vi "TimestampUpdate.vi"(10 "Timestamp":refnum<class "Timestamp.lvclass">, 11 "UserEvents":refnum<class "UserEvents.lvclass">) -> ()   [LabVIEW 2016]
uses:
  UserEvents/UserEvents.lvclass
  Common_RT_Timestamp/Timestamp/Timestamp.lvclass
  UserEvents/UserEvents.lvclass/UserEvents.ctl
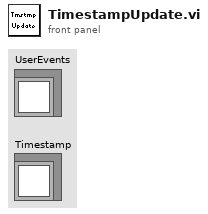
[diagram p1: front panel]
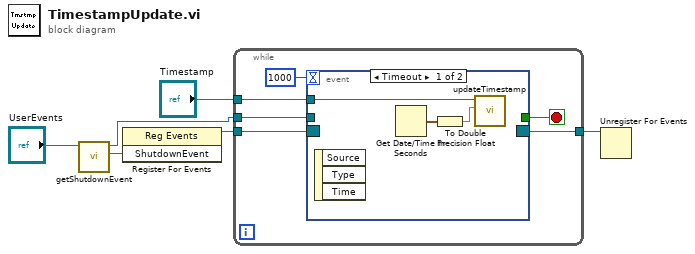
[diagram p0: block diagram]
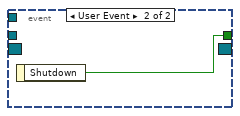
[diagram p2: hidden frame]
diagram:
  n1 = call "getShutdownEvent.vi"("UserEvents in"="UserEvents") -> ("ShutdownEvent"=w6:refnum<user-event>, "UserEvents out"=w4:refnum<class "UserEvents.lvclass">)  [unwired: 9 in]
  n2 = register-events(w6) -> (reference out=w5:refnum<event-registration>)  [unwired: 2 in, 1 out]
  n3 = while {
    tunnel: w5 -> [w11]
    tunnel: [w10] -> w3
    tunnel: w4 -> [w8]
    tunnel: "Timestamp" -> [w7]
    stop <- w9 stop-if-true
    n4 = event shown="[0] Timeout" {
      selector: w11 -> [_ _]
      dyn-events: [_ _] -> w10
      timeout: 1000 -> [_ _]
      tunnel: [_ w16] -> w9
      tunnel: w8 -> [_ _]
      tunnel: w7 -> [w15 _]
      event Timeout {
        n5 = event-data() -> ()  [unwired: 1 in, 3 out]
        n6 = Get Date/Time In Seconds() -> (seconds since 1Jan1904=w14:timestamp)
        n7 = To Double Precision Float(number=w14) -> (double precision float=w13:dbl)
        n8 = call "updateTimestamp.vi"("Timestamp"=w13, "Timestamp in"=w15) -> ()  [unwired: 8 in, 2 out]
      }
      event User Event {
        n9 = event-data() -> ("Shutdown"=w16:bool)  [unwired: 1 in]
      }
    }
  }
  n10 = Unregister For Events(event registration refnum=w3) -> ()  [unwired: 1 in, 1 out]
